vi "Remove U Folder.vi"() -> ()   [LabVIEW 2013]
panel:
  out "error out":errorcluster
  out "file or folder exists?":bool
  # "Used when SD card is not present"
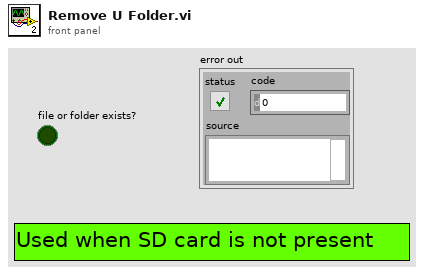
[diagram p1: front panel]
types:
  T1 = enum16{"open", "replace", "create", "open or create", "replace or create", "replace or create with confirmation"}
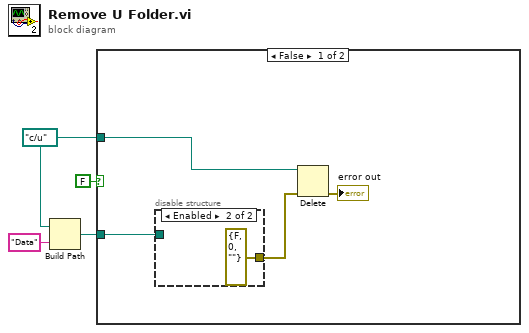
[diagram p0: block diagram]
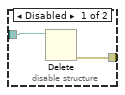
[diagram p2: hidden frame]
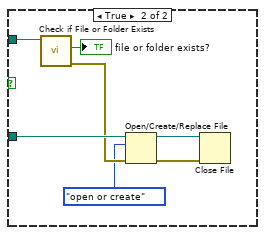
[diagram p3: hidden frame]
diagram:
  w3 = path "c:/u" ("path")
  n1 = Build Path(base path=w3, name or relative path="Data") -> (appended path=w1:path)
  n2 = case shown="False" FALSE {
    tunnel: w3 -> [w8 w17]
    tunnel: w1 -> [w6 w16]
    frame False {
      n3 = disable-structure shown="Enabled" {
        disable-tunnel: w6 -> [w10 _]
        disable-tunnel: [w9 errorcluster {"status"=FALSE, "code"=0, "source"=""} ("error out")] -> w5
        frame Disabled {
          n4 = Delete(path (use dialog)=w10) -> (error out=w9:errorcluster)  [unwired: 4 in, 2 out]
        }
        frame Enabled {
        }
      }
      n5 = Delete(path (use dialog)=w8, error in=w5) -> (error out=→"error out":errorcluster)  [unwired: 3 in, 2 out]
    }
    frame True {
      n6 = call <vilib>:"Check if File or Folder Exists.vi"("path"=w17) -> ("error out"=w13:errorcluster, "file or folder exists?"=→"file or folder exists?":bool)  [unwired: 8 in, 1 out]
      n7 = Open/Create/Replace File(file path (use dialog)=w16, error in=w13, operation (0:open)=T1."open or create") -> (refnum out=w15:refnum<file>, error out=w14:errorcluster)  [unwired: 3 in, 1 out]
      n8 = Close File(refnum=w15, error in=w14) -> ()  [unwired: 2 out]
    }
  }
